vi "Initiate Continuous.vi"(8 "error in (no error)":errorcluster, 10 "Initiate Continuous":bool, 11 "VISA resource name":refnum<visa-resource-name>) -> (0 "error out":errorcluster, 3 "VISA resource name out":refnum<visa-resource-name>)   [LabVIEW 2022 SP3, in "MagnaDC.lvlib"]
uses:
  MagnaDC.lvlib
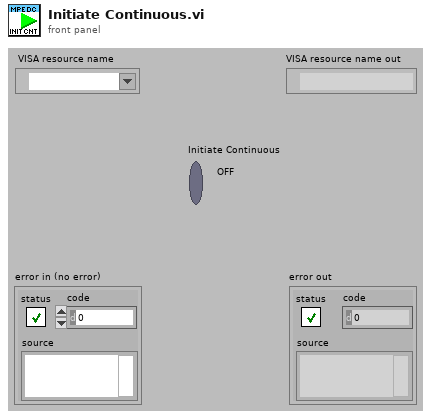
[diagram p1: front panel]
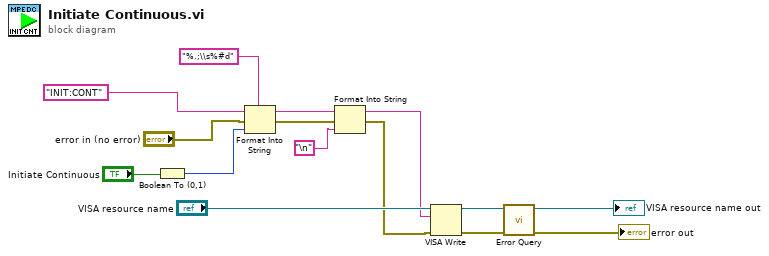
[diagram p0: block diagram]
diagram:
  n1 = Boolean To (0,1)(Boolean="Initiate Continuous") -> (0, 1=w3:i16)
  n2 = Format Into String(format string="%.;\\s%#d", initial string="INIT:CONT", error in="error in (no error)", w3) -> (resulting string=w4:string, error out=w5:errorcluster)
  n3 = Format Into String(initial string=w4, error in=w5, "\n") -> (resulting string=w8:string, error out=w7:errorcluster)  [unwired: 1 in]
  n4 = VISA Write(VISA resource name="VISA resource name", write buffer=w8, error in (no error)=w7) -> (VISA resource name out=w15:refnum<visa-resource-name>, error out=w14:errorcluster)  [unwired: 1 out]
  n5 = call "Error Query.vi"("error in (no error)"=w14, "VISA resource name"=w15) -> ("error out"=→"error out":errorcluster, "VISA resource name out"=→"VISA resource name out":refnum<visa-resource-name>)  [unwired: 6 in, 2 out]
